vi "Translational Align.vi"(11 "Robot Velocities In":cluster{"x":dbl, "y":dbl, "w":dbl}) -> (3 "Robot Velocities Out":cluster{"x":dbl, "y":dbl, "w":dbl})   [LabVIEW 2020]
uses:
  <vilib>/Rock Robotics/Network Tables/NT Read Number.vi
panel:
  out "Err/Out Chart":cluster{dbl, dbl}(graph)
  out "SP/PV Chart":cluster{"setpoint":dbl, "process variable":dbl}(graph)
  out "tx (error)":dbl
  # "s"
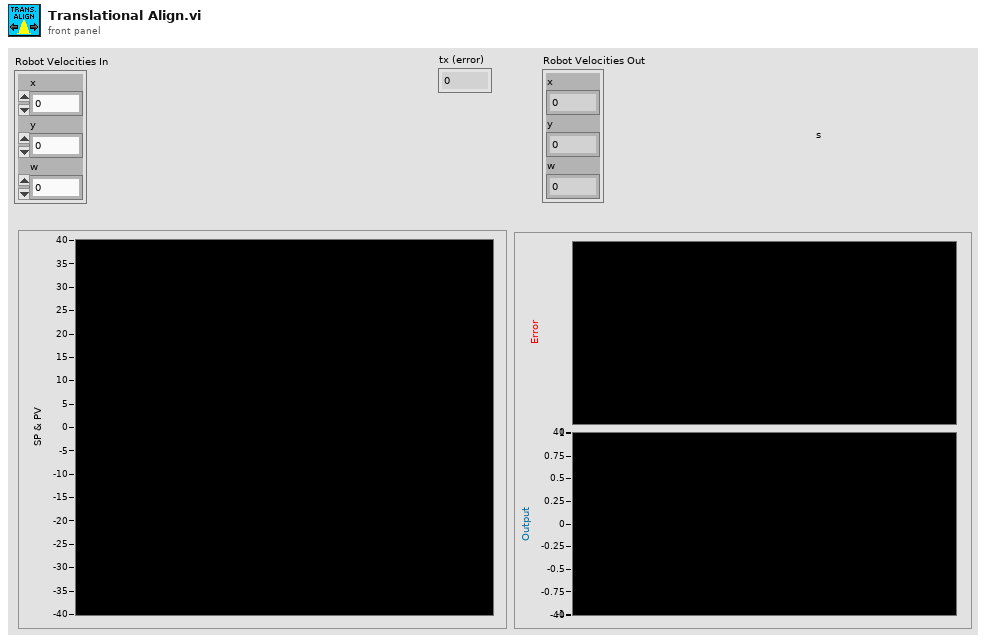
[diagram p1: front panel]
types:
  T1 = cluster{"proportional gain (Kp)":dbl, "integral time (Ki)":dbl, "derivative time (Kd)":dbl}
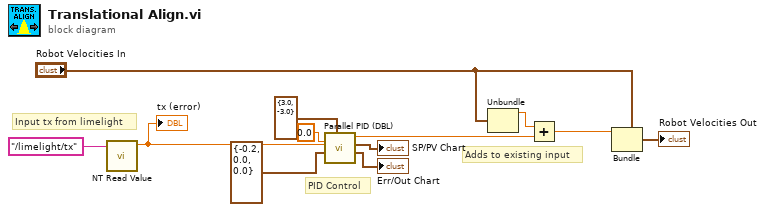
[diagram p0: block diagram]
diagram:
  # "Input tx from limelight"
  # "Adds to existing input"
  # "PID Control"
  n1 = call-poly <vilib>:"NT Read Value.vi"("name"="/limelight/tx") -> ("value"=w2:dbl)  [unwired: 8 in, 2 out]
  "tx (error)" <- w2
  n2 = call <vilib>:"Parallel PID (DBL).vi"("output range"=cluster{"high":dbl, "low":dbl} {"high"=3.0, "low"=-3.0}, "PID gains"=T1 {"proportional gain (Kp)"=-0.2, "integral time (Ki)"=0.0, "derivative time (Kd)"=0.0}, "process variable"=w2, "setpoint"=0.0) -> ("Err/Out Chart"=→"Err/Out Chart":cluster{dbl, dbl}, "SP/PV Chart"=→"SP/PV Chart":cluster{"setpoint":dbl, "process variable":dbl}, "output"=w6:dbl)  [unwired: 4 in, 1 out]
  n3 = Unbundle("Robot Velocities In") -> ("x"=w5:dbl)  [unwired: 2 out]
  n4 = Add(x=w5, y=w6) -> (x+y=w4:dbl)
  n5 = Bundle(cluster="Robot Velocities In", "x"=w4) -> (→"Robot Velocities Out":cluster{"x":dbl, "y":dbl, "w":dbl})  [unwired: 2 in]
